vi "Service Init.vi"(8 "error in (no error)":errorcluster, 9 "NIVS.Workspace Event":refnum<event-registration>, 10 "NIVS.Project File Path":path, 11 "NIVS.Gateway IP Address":string) -> (0 "error out":errorcluster, 3 "System Refs Cluster":T1, 4 "No CAN Logs":bool)   [LabVIEW 2010, in "CAN Log Transfer and Convert.lvlib"]
uses:
  CAN Log Transfer and Convert.lvlib
  Service Ref Cluster.ctl
  Queue Typedef.ctl
  <vilib>/NI Veristand/Execution/Workspace/WorkspaceAPI.ctl
  NationalInstruments.VeriStand.ClientAPI
  <vilib>/NI Veristand/Execution/Stimulus/StimulusAPI.ctl
  <vilib>/NI Veristand/Execution/Workspace/SystemStateRegEventRef.ctl
  <vilib>/NI Veristand/Execution/Workspace/SystemStateEventRef.ctl
  CAN Sysdef Data.ctl
  Stop FGV Commands.ctl
  Qd Functional Global Action.ctl
  <vilib>/NI Veristand/Execution/Workspace/NI_VS Workspace ExecutionAPI.lvlib
  <vilib>/NI Veristand/Execution/Stimulus/NI_VS Stimulus ExecutionAPI.lvlib
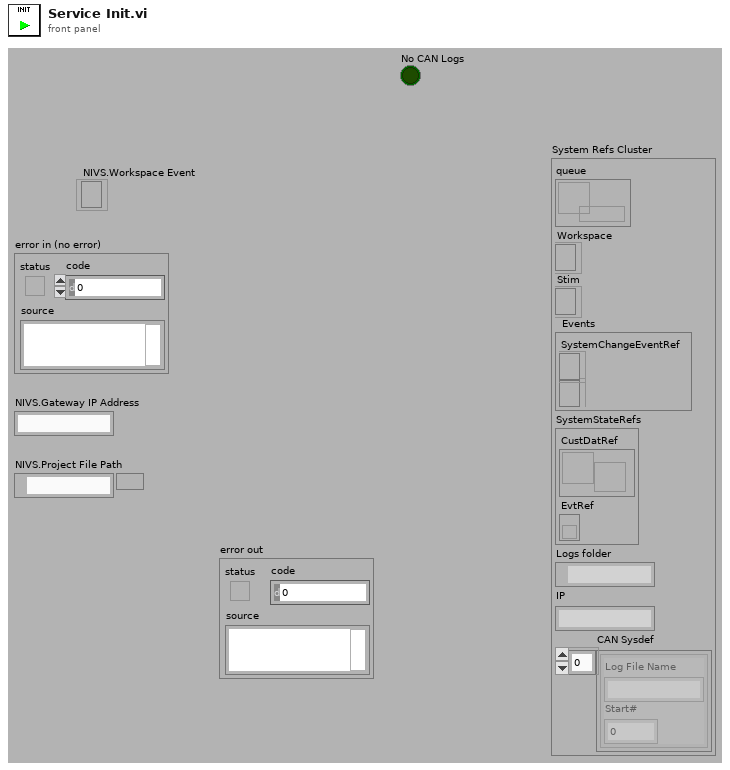
[diagram p1: front panel]
types:
  T1 = typedef "CAN Log Transfer and Convert.lvlib/Service Ref Cluster.ctl" = cluster{"queue":refnum<queue>, "Workspace":T2, "Stim":T3, "Events":cluster{"SystemChangeEventRef":T4, "NIVS.Workspace Event":refnum<event-registration>}, "SystemStateRefs":T5, "Logs folder":path, "IP":string, "CAN Sysdef":T6[]}
  T2 = typedef "NI_VS Workspace ExecutionAPI.lvlib/WorkspaceAPI.ctl" = refnum<k24>
  T3 = typedef "NI_VS Stimulus ExecutionAPI.lvlib/StimulusAPI.ctl" = refnum<k24>
  T4 = typedef "NI_VS Workspace ExecutionAPI.lvlib/SystemStateRegEventRef.ctl" = refnum<event-registration>
  T5 = typedef "NI_VS Workspace ExecutionAPI.lvlib/SystemStateEventRef.ctl" = cluster{"CustDatRef":refnum<user-event>, "EvtRef":refnum<k27>}
  T6 = typedef "CAN Log Transfer and Convert.lvlib/CAN Sysdef Data.ctl" = cluster{"Log File Name":string, "Start#":u16}
  T7 = typedef "CAN Log Transfer and Convert.lvlib/Qd Functional Global Action.ctl" = enum16{"Incr", "Reset", "Get"}
  T8 = typedef "CAN Log Transfer and Convert.lvlib/Queue Typedef.ctl" = cluster{"Path":path, "CAN Logs":string[]}
  T9 = typedef "CAN Log Transfer and Convert.lvlib/Stop FGV Commands.ctl" = enum16{"Write", "Read", "Reset"}
  T10 = cluster{"SystemChangeEventRef":T4, "NIVS.Workspace Event":refnum<event-registration>}
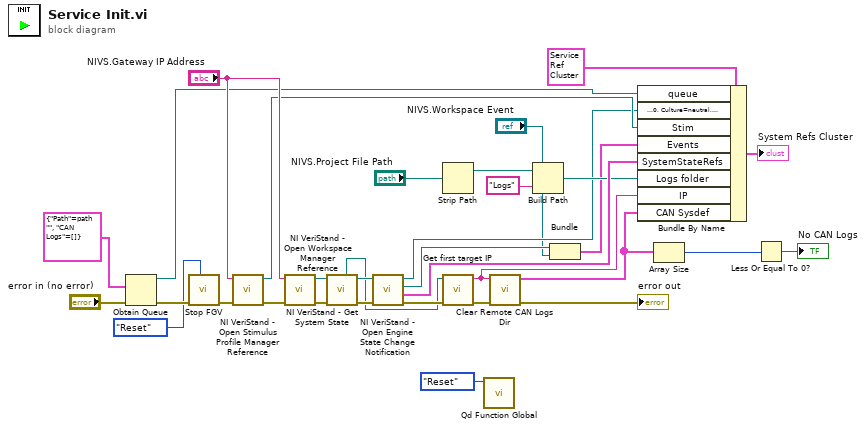
[diagram p0: block diagram]
diagram:
  n1 = Obtain Queue(element data type=T8 {"Path"=path "", "CAN Logs"=[]} ("Queue Data"), error in (no error)="error in (no error)") -> (queue out=w18:refnum<queue>, error out=w33:errorcluster)  [unwired: 3 in, 1 out]
  n2 = call "Stop FGV.vi"("Command"=Stop_FGV_Commands."Reset", "error in (no error)"=w33) -> ("error out"=w31:errorcluster)  [unwired: 7 in, 2 out]
  n3 = call <vilib>:"NI VeriStand - Open Stimulus Profile Manager Reference.vi"("error in (no error)"=w31, "Gateway IP Address (\"\": localhost)"="NIVS.Gateway IP Address") -> ("error out"=w25:errorcluster, "StimulusProfileManager"=w23:T3)  [unwired: 8 in]
  n4 = call <vilib>:"NI VeriStand - Open Workspace Manager Reference.vi"("error in (no error)"=w25, "Gateway IP Address (\"\": localhost)"="NIVS.Gateway IP Address") -> ("error out"=w15:errorcluster, "WorkspaceManager"=w14:T2)  [unwired: 8 in]
  n5 = call <vilib>:"NI VeriStand - Get System State.vi"("error in (no error)"=w15, "WorkspaceManager in"=w14) -> ("error out"=w13:errorcluster, "WorkspaceManager  out"=w12:T2, "System Definition File"=w11:path)  [unwired: 5 in, 2 out]
  n6 = call <vilib>:"NI VeriStand - Open Engine State Change Notification.vi"("error in (no error)"=w13, "WorkspaceManager in"=w12) -> ("error out"=w17:errorcluster, "SystemStateRefs"=w22:T5, "SystemChangeEventRef"=w8:T4, "WorkspaceManager out"=w16:T2)  [unwired: 6 in]
  n7 = Strip Path(path="NIVS.Project File Path") -> (stripped path=w27:path)  [unwired: 1 out]
  n8 = call "Get first target IP.vi"("error in (no error)"=w17, "System Definition File"=w11) -> ("error out"=w5:errorcluster, "IPAddress"=w4:string)  [unwired: 8 in]
  n9 = call "Qd Function Global.vi"("Action"=Qd_Functional_Global_Action."Reset") -> ()  [unwired: 10 in, 1 out]
  n10 = call "Clear Remote CAN Logs Dir.vi"("error in (no error)"=w5, "address"=w4) -> ("error out"=→"error out":errorcluster, "Logs To Transfer"=w2:T6[])  [unwired: 8 in]
  n11 = Build Path(base path=w27, name or relative path="Logs") -> (appended path=w21:path)
  n12 = Bundle("SystemChangeEventRef"=w8, "NIVS.Workspace Event"="NIVS.Workspace Event") -> (w6:T10)  [unwired: 1 in]
  n13 = Bundle By Name(cluster=T1 {"queue"=refnum, "Workspace"=refnum, "Stim"=refnum, "Events"={"SystemChangeEventRef"=refnum, "NIVS.Workspace Event"=refnum}, "SystemStateRefs"={"CustDatRef"=refnum, "EvtRef"=refnum}, "Logs folder"=path "", "IP"="", "CAN Sysdef"=[]} ("Service Refs Cluster"), "queue"=w18, "Workspace"=w16, "Stim"=w23, "Events"=w6, "SystemStateRefs"=w22, "Logs folder"=w21, "IP"=w4, "CAN Sysdef"=w2) -> (→"System Refs Cluster":T1)
  n14 = Array Size(array=w2) -> (size(s)=w10:i32)
  n15 = Less Or Equal To 0?(x=w10) -> (x <= 0?=→"No CAN Logs":bool)
